vi "LogCreate.vi"(7 "Application Configuration":T2={"DUT"={"Count"=1, "Wirings"=[], "Names"=[]}, "Log"={"Start"={"Trigger Type"=enum."Immediate", "Timer (sec)"=0.0, "Digital IO Line"=0, "Digital IO Edge"=enum."Rising"}, "Rollover"={"Trigger Type"=enum."None", "Timer (sec)"=0.0, "File Size (MB)"=0, "Digital IO Line"=0, "Digital IO Edge"=enum."Rising"}, "Stop"={"Trigger Type"=enum."None", "Timer (sec)"=0.0, "File Size (MB)"=0, "Digital IO Line"=0, "Digital IO Edge"=enum."Rising"}}, "Trigger"={"Input"={"Type"=enum."None", "Timeout (ms)"=0, "Delay (ms)"=0, "Digital IO Line (1-14)"=0, "Digital IO Mode"=enum."Falling"}, "Output"={"Type"=enum."None", "Delay (ms)"=0, "Digital IO Line (1-14)"=0, "Digital IO Mode"=enum."Falling", "Digital IO Pulse Width (sec)"=0.0}}, "Sources"=[], "Measures"=[]} {"Measures"."Count" min=1 step=1; "Trigger"."Output"."Digital IO Line (1-14)" min=1 max=14 step=1}, 8 "Error In":errorcluster, 11 "Executable Configuration":T1) -> (0 "Error Out":errorcluster, 3 "Log File":path)   [LabVIEW 2012]
uses:
  Setup.ctl
  DUTConfiguration.ctl
  driver/Public/Controls/SMUSense.ctl
  LogConfiguration.ctl
  LogStartConfiguration.ctl
  LogStartTriggerType.ctl
  LogDigitalIOTriggerEdge.ctl
  LogRolloverConfiguration.ctl
  LogRolloverTriggerType.ctl
  LogStopConfiguration.ctl
  LogStopTriggerType.ctl
  TriggerConfiguration.ctl
  TriggerInputConfiguration.ctl
  TriggerInputType.ctl
  driver/Public/Controls/TriggerMode.ctl
  TriggerOutputConfiguration.ctl
  TriggerOutputType.ctl
  SourceConfiguration.ctl
  SourceFunction.ctl
  MeasureConfiguration.ctl
  ExecutableConfiguration.ctl
  LogFileGlobalAction.ctl
  LogStartTimeGlobalAction.ctl
  libs/LV-Utilities/LV-Utilities.lvlib
  driver/Keithley-2602.lvlib
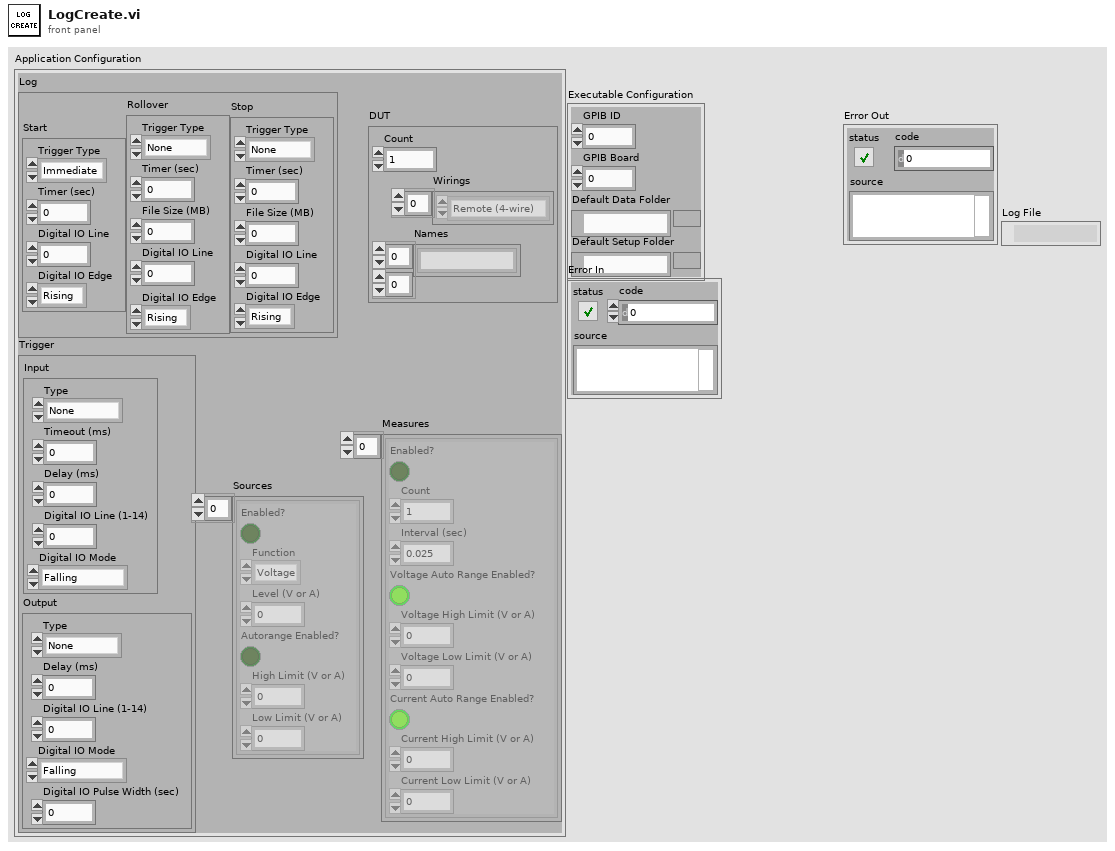
[diagram p1: front panel]
types:
  T1 = typedef "ExecutableConfiguration.ctl" = cluster{"GPIB ID":u8, "GPIB Board":u8, "Default Data Folder":path, "Default Setup Folder":path}
  T2 = typedef "Setup.ctl" = cluster{"DUT":T3, "Log":T5, "Trigger":T13, "Sources":T19[], "Measures":T21[]}
  T3 = typedef "DUTConfiguration.ctl" = cluster{"Count":u32, "Wirings":T4[], "Names":string[][]}
  T4 = typedef "Keithley-2602.lvlib/SMUSense.ctl" = enum16{"Local (2-wire)", "Remote (4-wire)", "Calibration"}
  T5 = typedef "LogConfiguration.ctl" = cluster{"Start":T6, "Rollover":T9, "Stop":T11}
  T6 = typedef "LogStartConfiguration.ctl" = cluster{"Trigger Type":T7, "Timer (sec)":dbl, "Digital IO Line":u8, "Digital IO Edge":T8}
  T7 = typedef "LogStartTriggerType.ctl" = enum16{"Immediate", "User", "Timer", "Digital IO"}
  T8 = typedef "LogDigitalIOTriggerEdge.ctl" = enum16{"Rising", "Falling"}
  T9 = typedef "LogRolloverConfiguration.ctl" = cluster{"Trigger Type":T10, "Timer (sec)":dbl, "File Size (MB)":u32, "Digital IO Line":u8, "Digital IO Edge":T8}
  T10 = typedef "LogRolloverTriggerType.ctl" = enum16{"None", "Timer", "File Size", "Digital IO"}
  T11 = typedef "LogStopConfiguration.ctl" = cluster{"Trigger Type":T12, "Timer (sec)":dbl, "File Size (MB)":u32, "Digital IO Line":u8, "Digital IO Edge":T8}
  T12 = typedef "LogStopTriggerType.ctl" = enum16{"None", "User", "Timer", "File Size", "Digital IO"}
  T13 = typedef "TriggerConfiguration.ctl" = cluster{"Input":T14, "Output":T17}
  T14 = typedef "TriggerInputConfiguration.ctl" = cluster{"Type":T15, "Timeout (ms)":u32, "Delay (ms)":u32, "Digital IO Line (1-14)":u8, "Digital IO Mode":T16}
  T15 = typedef "TriggerInputType.ctl" = enum16{"None", "Digital IO", "Bus"}
  T16 = typedef "Keithley-2602.lvlib/TriggerMode.ctl" = enum16{"Falling", "Rising", "Either", "Synchronous"}
  T17 = typedef "TriggerOutputConfiguration.ctl" = cluster{"Type":T18, "Delay (ms)":u32, "Digital IO Line (1-14)":u8, "Digital IO Mode":T16, "Digital IO Pulse Width (sec)":dbl}
  T18 = typedef "TriggerOutputType.ctl" = enum16{"None", "Digital IO", "Bus"}
  T19 = typedef "SourceConfiguration.ctl" = cluster{"Enabled?":bool, "Function":T20, "Level (V or A)":dbl, "Autorange Enabled?":bool, "High Limit (V or A)":dbl, "Low Limit (V or A)":dbl}
  T20 = typedef "SourceFunction.ctl" = enum16{"Voltage", "Current"}
  T21 = typedef "MeasureConfiguration.ctl" = cluster{"Enabled?":bool, "Count":u8, "Interval (sec)":dbl, "Voltage Auto Range Enabled?":bool, "Voltage High Limit (V or A)":dbl, "Voltage Low Limit (V or A)":dbl, "Current Auto Range Enabled?":bool, "Current High Limit (V or A)":dbl, "Current Low Limit (V or A)":dbl}
  T22 = typedef "LogStartTimeGlobalAction.ctl" = enum16{"Set", "Get"}
  T23 = typedef "LogFileGlobalAction.ctl" = enum16{"Open", "Write", "Size", "Close"}
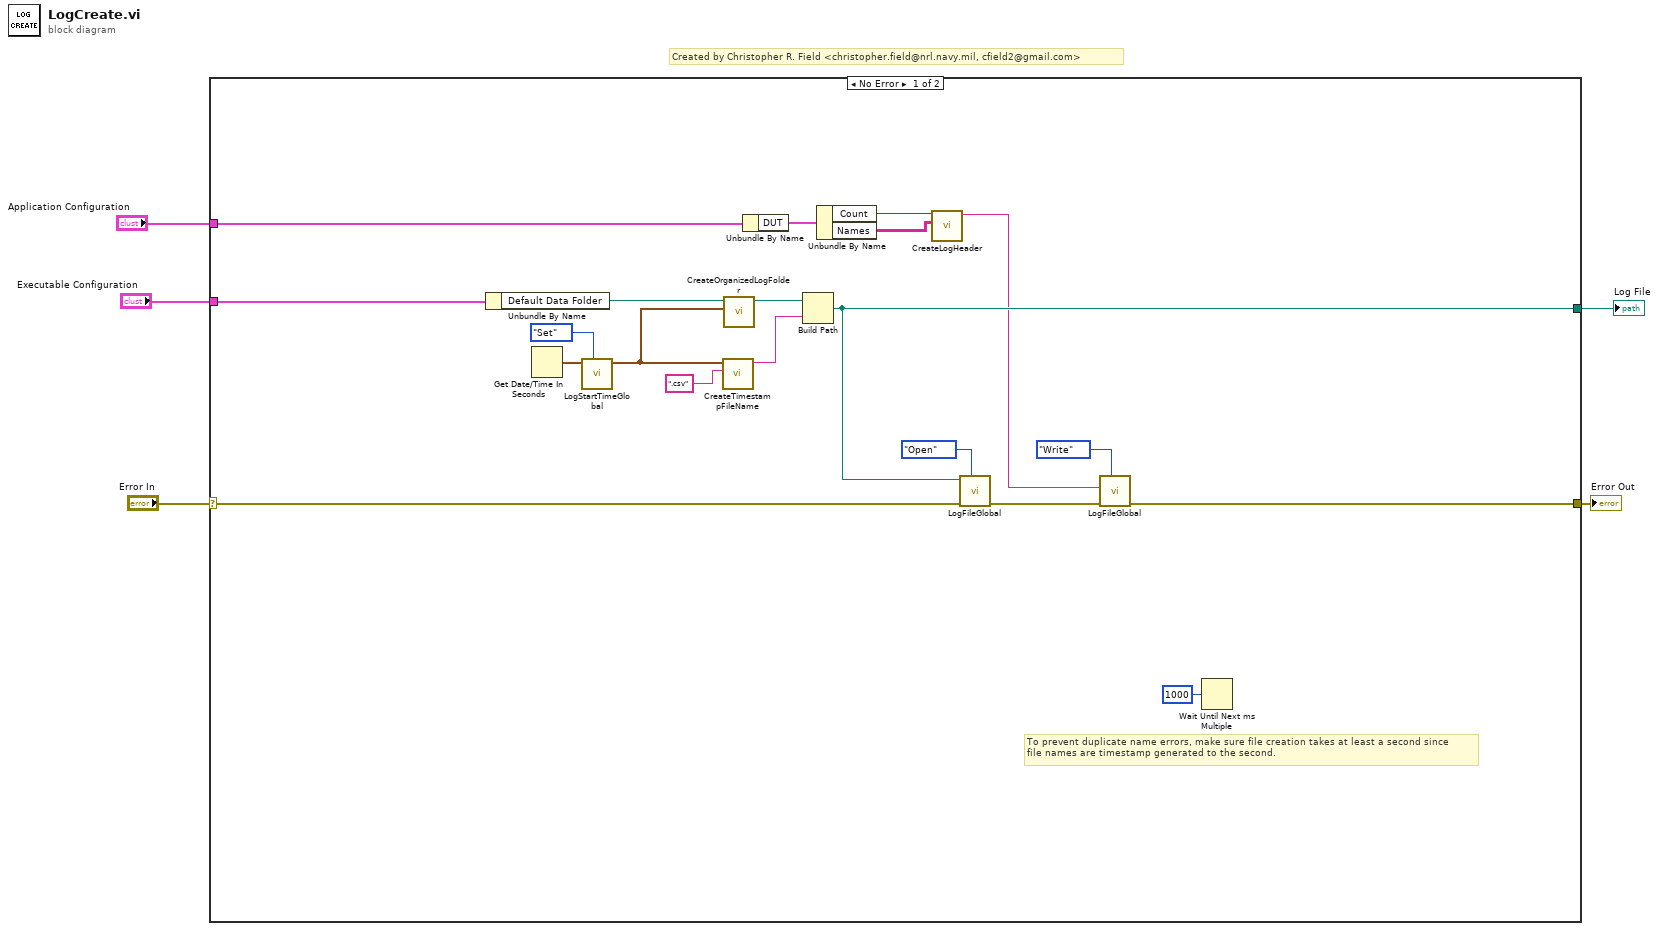
[diagram p0: block diagram]
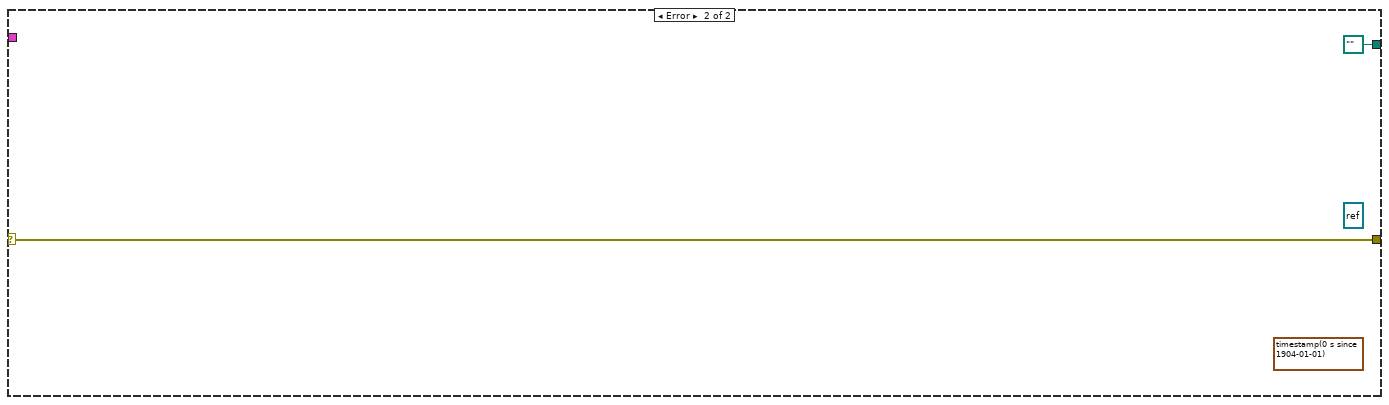
[diagram p2: hidden frame]
diagram:
  # "Created by Christopher R. Field <christopher.field@nrl.navy.mil, cfield2@gmail.com>"
  n1 = case shown="No Error" "Error In" {
    selector: "Error In" -> [w9 w27]
    tunnel: "Executable Configuration" -> [w21 _]
    tunnel: [w10 w27] -> w3
    tunnel: "Application Configuration" -> [w20 _]
    tunnel: [w14 path "" ("appended path")] -> w1
    frame No Error {
      # "To prevent duplicate name errors, make sure file creation takes at least a second since\nfile names are timestamp generated to the second."
      n2 = Unbundle By Name(w21) -> ("Default Data Folder"=w22:path)
      n3 = Get Date/Time In Seconds() -> (seconds since 1Jan1904=w7:timestamp)
      n4 = call "LogStartTimeGlobal.vi"("Action"=LogStartTimeGlobalAction."Set", "Set Value"=w7) -> ("Value Out"=w6:timestamp)  [unwired: 9 in]
      n5 = call "CreateTimestampFileName.vi"("File Extension (.csv)"=".csv", "Time Stamp"=w6) -> ("Timestamp File Name"=w23:string)  [unwired: 9 in]
      n6 = call "CreateOrganizedLogFolder.vi"("Time Stamp"=w6, "Base Log Path"=w22) -> ("Organized Log Path"=w24:path)  [unwired: 8 in, 1 out]
      n7 = Unbundle By Name(w20) -> ("DUT"=w19:T3)
      n8 = Build Path(base path=w24, name or relative path=w23) -> (appended path=w14:path)
      n9 = Unbundle By Name(w19) -> ("Count"=w18:u32, "Names"=w17:string[][])
      n10 = call "CreateLogHeader.vi"("Names"=w17, "DUT Count"=w18) -> ("Column Headers"=w12:string)  [unwired: 9 in]
      n11 = call "LogFileGlobal.vi"("Action"=LogFileGlobalAction."Open", "Error In"=w9, "Path"=w14) -> ("Error Out"=w13:errorcluster)  [unwired: 7 in, 1 out]
      n12 = call "LogFileGlobal.vi"("Action"=LogFileGlobalAction."Write", "Error In"=w13, "CSV String"=w12) -> ("Error Out"=w10:errorcluster)  [unwired: 7 in, 1 out]
      n13 = Wait Until Next ms Multiple(millisecond multiple=u32 1000) -> ()  [unwired: 1 out]
    }
    frame Error {
      (unwired) timestamp(0 s since 1904-01-01) ("seconds since 1Jan1904")
      (unwired) refnum<file> refnum ("refnum out")
    }
  }
  "Error Out" <- w3
  "Log File" <- w1
